vi "Clip AO Waveforms.vi"(8 "error in (no error)":errorcluster, 10 "AO []":waveform(dbl)[](array[waveform]), 11 "Lockin.DAQ in":refnum<class "Lockin.DAQ.lvclass">) -> (0 "error out":errorcluster, 2 "Clipped AO []":waveform(dbl)[](array[waveform]), 3 "Lockin.DAQ out":refnum<class "Lockin.DAQ.lvclass">)   [LabVIEW 2016, in "Lockin.DAQ.lvclass"]
uses:
  Lockin.DAQ.lvclass
  Lockin.DAQ.lvclass/Lockin.DAQ.ctl
  Instrument.Lockin/Instrument.Lockin.lvclass
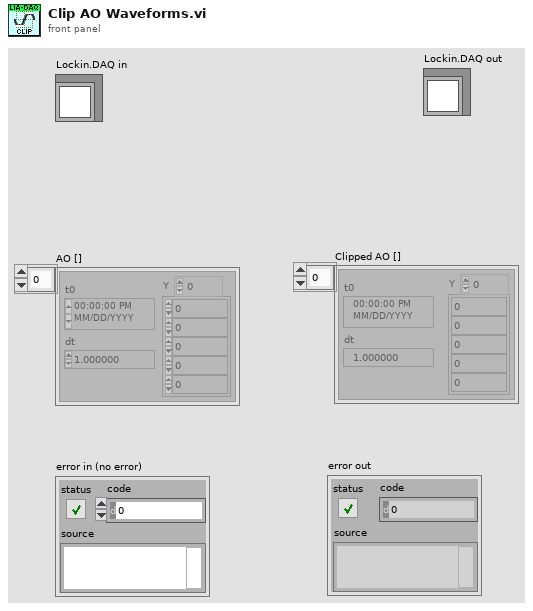
[diagram p1: front panel]
types:
  T1 = typedef "Lockin.DAQ.lvclass/AO.config-array.ctl" = T2[]
  T2 = typedef "Lockin.DAQ.lvclass/AO.config-cluster.ctl" = cluster{"AO.channels":tag, "AO.Range":T3, "output terminal configuration":i32, "DAQ Type":T4}
  T3 = typedef "Lockin.DAQ.lvclass/446xAO-enum.ctl" = enum16{"±0.1", "±1.0", "±10.0"}
  T4 = typedef "Lockin.DAQ.lvclass/DAQType-enum.ctl" = enum16{"None", "USB 4431", "PXI 446x"}
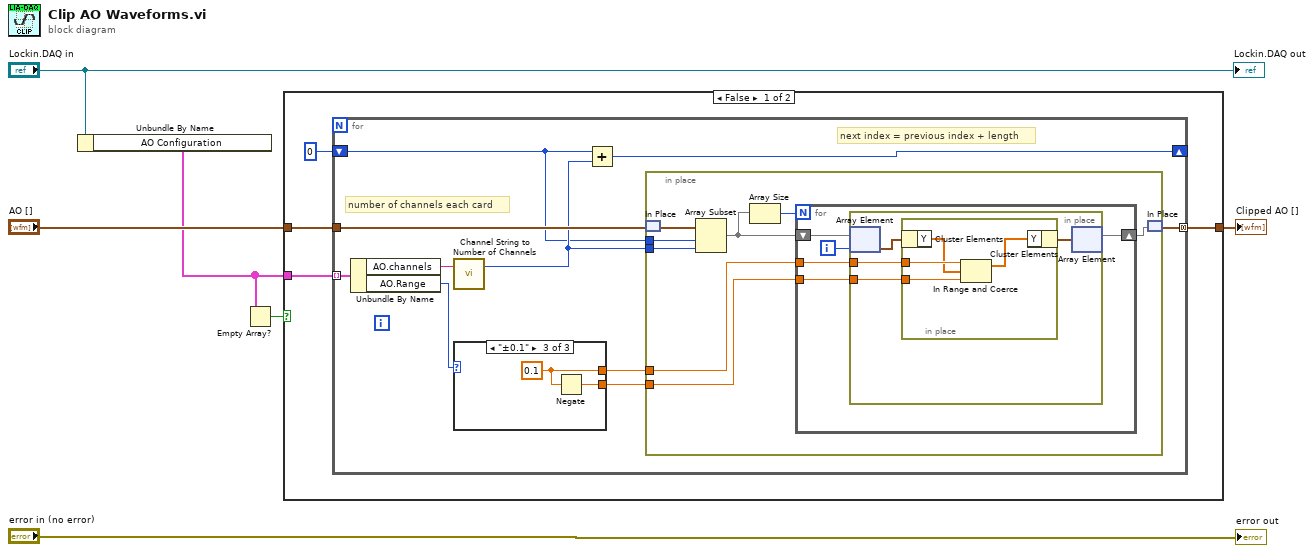
[diagram p0: block diagram]
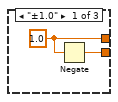
[diagram p2: hidden frame]
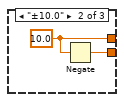
[diagram p3: hidden frame]
diagram:
  n1 = Unbundle By Name("Lockin.DAQ in") -> ("AO Configuration"=w1:T1)
  n2 = Empty Array?(array=w1) -> (empty?=w3:bool)
  n3 = case shown="False" w3 {
    tunnel: [w10 w48] -> w6
    tunnel: "AO []" -> [w9 w48]
    tunnel: w1 -> [w8 _]
    frame False {
      n4 = for {
        tunnel: w8 -> [w20] mode=indexing
        tunnel: w9 -> [w14]
        tunnel: [w15] -> w10 mode=concatenating
        shift-right: [w13] -> _
        shift-left: 0 -> [w11]
        # "next index = previous index + length"
        # "number of channels each card"
        n5 = Unbundle By Name(w20) -> ("AO.channels"=w17:tag, "AO.Range"=w16:T3)
        n6 = call "Channel String to Number of Channels.vi"("Channels String"=w17) -> ("# channels"=w12:i32)  [unwired: 2 in]
        n7 = case shown="\"±0.1\"" w16 {
          tunnel: [w43 w45 w47] -> w19
          tunnel: [w42 w44 w46] -> w18
          frame "±1.0" {
            w43 = 1.0
            n8 = Negate(x=w43) -> (-x=w42:dbl)
          }
          frame "±10.0" {
            w45 = 10.0
            n9 = Negate(x=w45) -> (-x=w44:dbl)
          }
          frame "±0.1" {
            w47 = 0.1
            n10 = Negate(x=w47) -> (-x=w46:dbl)
          }
        }
        n11 = Add(x=w11, y=w12) -> (x+y=w13:i32)
        n12 = in-place {
          in-place-border: w12 -> [w28]
          in-place-border: w11 -> [w27]
          in-place-border: w19 -> [w26]
          in-place-border: w18 -> [w25]
          n13 = in-place-match #1(w14) -> (w24:waveform(dbl)[])
          n14 = Array Subset(array=w24, index=w27, length=w28) -> (w21:waveform(dbl)[])
          n15 = Array Size(array=w21) -> (size(s)=w22:i32)
          n16 = for {
            N: w22 -> [_]
            tunnel: w26 -> [w33]
            tunnel: w25 -> [w32]
            shift-right: [w29] -> w23
            shift-left: w21 -> [w30]
            i -> [w31]
            n17 = in-place {
              in-place-border: w33 -> [w37]
              in-place-border: w32 -> [w36]
              n18 = in-place-array #2(w30, w31) -> (w35:waveform(dbl))
              n19 = in-place {
                in-place-border: w37 -> [w41]
                in-place-border: w36 -> [w40]
                n20 = in-place-cluster #3(w35) -> ("Y"=w39:dbl[])
                n21 = In Range and Coerce(upper limit=w41, x=w39, lower limit=w40) -> (coerced(x)=w38:dbl[])  [unwired: 1 out]
                n22 = in-place-cluster #3("Y"=w38) -> (w34:waveform(dbl))
              }
              n23 = in-place-array #2(w34) -> (w29:waveform(dbl)[])  [unwired: 1 out]
            }
          }
          n24 = in-place-match #1(w23) -> (w15:waveform(dbl)[])
        }
      }
    }
    frame True {
      # "If AO Config = empty, do nothing"
    }
  }
  "Clipped AO []" <- w6
  "error out" <- "error in (no error)"
  "Lockin.DAQ out" <- "Lockin.DAQ in"
